vi "FRIC_navX_Internal_Serial_ProcessingLoop.vi"(7 "Device Number":T3, 11 "Rate (4Hz-200Hz)":u8=50 min=4 max=200) -> ()   [LabVIEW 2016]
doc: "This navX VI handles the reading/writing for the navX. All of the good stuff is in here.\nTHIS VI SHOULD NOT BE CALLED BY THE USER!"
uses:
  <vilib>/Rock Robotics/SystemInterfaces/i2clib/i2c_bus.ctl
  TypeDefs/Z900_navX_ProtocolTypeDef.ctl
  navX Library v2.lvlib
  TypeDefs/FRIC_navX_ProcessingLoopStatesTypeDef_I2C.ctl
  TypeDefs/Z900_navX_IntegrationControlRegisters.ctl
  TypeDefs/Z900_navX_ActionTypeDef.ctl
  TypeDefs/Z900_navX_NotifyPacketTypeDef.ctl
  TypeDefs/FRIC_navX_I2C Process Loop TypeDef.ctl
  <vilib>/Rock Robotics/SystemInterfaces/spilib/spi_bus.ctl
  <vilib>/Rock Robotics/WPI/SPI/WPI_SPIDevRef.ctl
  TypeDefs/Z900_navX_SerialStreamTypeDef.ctl
  <vilib>/Rock Robotics/WPI/SerialPort/WPI_SerialPortRef.ctl
  TypeDefs/FRIC_navX_DeviceNumbersTypeDef.ctl
  <vilib>/Rock Robotics/WPI/SerialPort/WPI_SerialPort.ctl
  <vilib>/Platform/TimedLoop/XDataNode/wakeup.ctl
  <vilib>/Platform/TimedLoop/XDataNode/XDNodeRunTimeDep.lvlib
  <vilib>/Platform/TimedLoop/XDataNode/nitl_modes.ctl
  <vilib>/Platform/TimedLoop/XDataNode/timing_clust.ctl
  <vilib>/Platform/TimedLoop/XDataNode/XDataNode.xnode
  <vilib>/ptbypt/NI_PtbyPt.lvlib
  TypeDefs/Z900_navX_DeviceTypeDef.ctl
panel:
  in  "Tab Control":enum32{"Page 1", "Page 2"}(tab)
  in  "Halt":bool
  out "Connected":bool
  out "error":errorcluster
  in  "Stream Type":T1=enum."AHRSAndPositioning"
  in  "Serial Port":T2=enum."MXP TTL"
  out "Loop Time":dbl format="%#.1g"
  out "Loop dt":i64
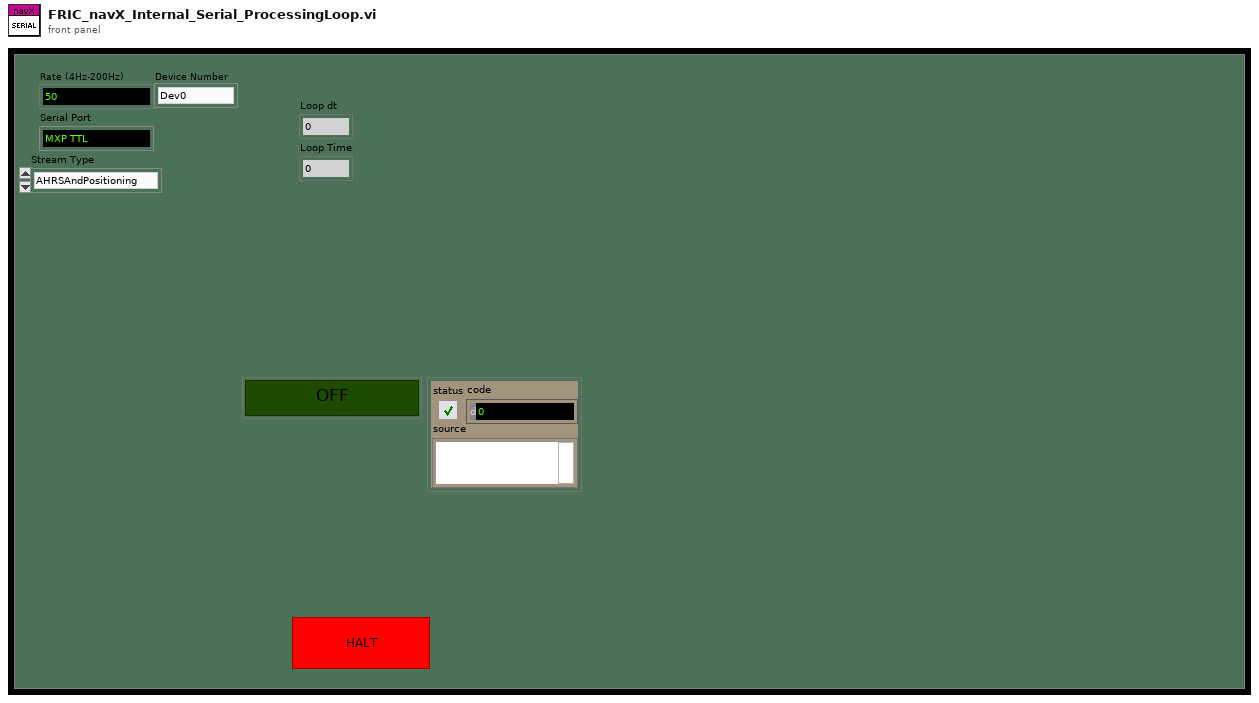
[diagram p1: front panel]
types:
  T1 = typedef "navX Library v2.lvlib/Z900_navX_SerialStreamTypeDef.ctl" = enum16{"YRPH", "Quaterinons", "Gyro/Raw", "AHRS", "AHRSAndPositioning"}
  T2 = typedef "WPI_SerialPort.ctl" = enum16{"Onboard RS-232", "MXP TTL", "USB 1", "USB 2"}
  T3 = typedef "FRIC_navX_DeviceNumbersTypeDef.ctl" = enum16{"Dev0", "Dev1", "Dev2", "Dev3"}
  T4 = typedef "FRIC_navX_I2C Process Loop TypeDef.ctl" = cluster{"State Array":T5[], "error":errorcluster, "FPGA Cluster":cluster{"Last Valid FPGA Time":dbl, "Error Count":i32, "Initialized":bool}, "Device Info":T6, "I2CDevRef":cluster{"DevStatus":errorcluster, "Device Address":u8, "Handle":i32, "I2C Bus":T8}, "Registry":u8[], "Command Array":T9[], "Connected?":bool, "navX Device Memory Size":i32, "notification":T10, "Memory Size Set":bool, "SPIDevRef":T12, "navX Serial Open":cluster{"Stream Type":T1, "Serial Port":T2}, "SerialPortRef":T14, "Serial Read Buffer":string, "Serial Write Buffer":string[], "Device Number":T3, "navX SPI Open":cluster{"SPI Bus":T13, "Clock Rate (Hz)":dbl}, "Loop dt":i64, "current time":timestamp, "Loop Time":i64}
  T5 = typedef "FRIC_navX_ProcessingLoopStatesTypeDef_I2C.ctl" = enum16{"Process", "INI", "Check Packets Valid", "Close", "Flush Serial", "Generate Command", "Last Packet Valid", "Open", "Read", "Reset Serial", "Set Termination Char", "Update AE", "Wait", "Write", "Exit"}
  T6 = typedef "navX Library v2.lvlib/Z900_navX_DeviceTypeDef.ctl" = cluster{"Interface":cluster{"Protocol":T7, "Update Rate (4Hz-100Hz)":u8, "navX Open TypeDef":variant}, "Notify Packet":refnum<notifier>, "Loop VI Refnum":refnum<vi>, "Ready to Close Occurrence Refnum":refnum<k4>}
  T7 = typedef "navX Library v2.lvlib/Z900_navX_ProtocolTypeDef.ctl" = enum16{"SERIAL", "I2C", "SPI"}
  T8 = typedef "i2c_bus.ctl" = enum16{"I2C On-Board", "I2C MXP", "Invalid"}
  T9 = typedef "navX Library v2.lvlib/Z900_navX_IntegrationControlRegisters.ctl" = u8
  T10 = typedef "navX Library v2.lvlib/Z900_navX_NotifyPacketTypeDef.ctl" = cluster{"navX Action":T11, "Data":variant}
  T11 = typedef "navX Library v2.lvlib/Z900_navX_ActionTypeDef.ctl" = enum16{"None", "Halt", "Update Serial Protocol", "Zero-Yaw", "Zero-Displacement", "Zero-Velocity"}
  T12 = typedef "WPI_SPIDevRef.ctl" = cluster{"DevStatus":errorcluster, "Handle":i32, "SPI Bus":T13}
  T13 = typedef "spi_bus.ctl" = enum16{"SPI On-Board, CS0", "SPI On-Board, CS1", "SPI On-Board, CS2", "SPI On-Board, CS3", "SPI MXP", "Invalid"}
  T14 = typedef "WPI_SerialPortRef.ctl" = cluster{"DevStatus":errorcluster, "Serial Port Name":refnum<visa-resource-name>}
  T15 = typedef "XDNodeRunTimeDep.lvlib/timing_clust.ctl" = cluster{"Expected End [f-1]":u64, "Actual End [f-1]":u64, "Finished Late? [f-1]":bool, "Expected End [i-1]":u64, "Actual End [i-1]":u64, "Finished Late? [i-1]":bool, "Expected Start [i]":u64, "Actual Start [i]":u64, "Expected Start [f]":u64, "Actual Start [f]":u64, "Source Name":string, "Structure Name":string, "Period":i64, "Deadline":i64, "Offset":i64, "Start":i64, "Priority":i32, "Timeout":i32, "Mode":T16, "Wakeup Reason":T17, "Error":errorcluster, "Source Type":string, "Secondary Source Type":string, "Global End Time":u64, "Global Start Time":u64, "Frame Duration":u64, "Iteration Duration":u64, "Assigned CPU":i32, "I/O Scan Engine Mode":u32}
  T16 = typedef "XDNodeRunTimeDep.lvlib/nitl_modes.ctl" = enum32{"No Change", "Process missed periods, maintain original phase", "Discard missed periods, maintain original phase", "Process missed periods, ignore original phase", "Discard missed periods, ignore original phase"}
  T17 = typedef "XDNodeRunTimeDep.lvlib/wakeup.ctl" = enum32{"Normal", "Aborted", "Asynchronous wakeup", "Timing source error", "Timed loop error", "Timeout"}
  T18 = typedef "Z900_navX_ActionTypeDef.ctl" = enum16{"None", "Halt", "Normal Read", "Update Serial Protocol", "Update Rate Htz", "Zero-Yaw", "Zero-Displacement", "Zero-Velocity"}
  T19 = cluster{"Last Valid FPGA Time":dbl, "Error Count":i32, "Initialized":bool}
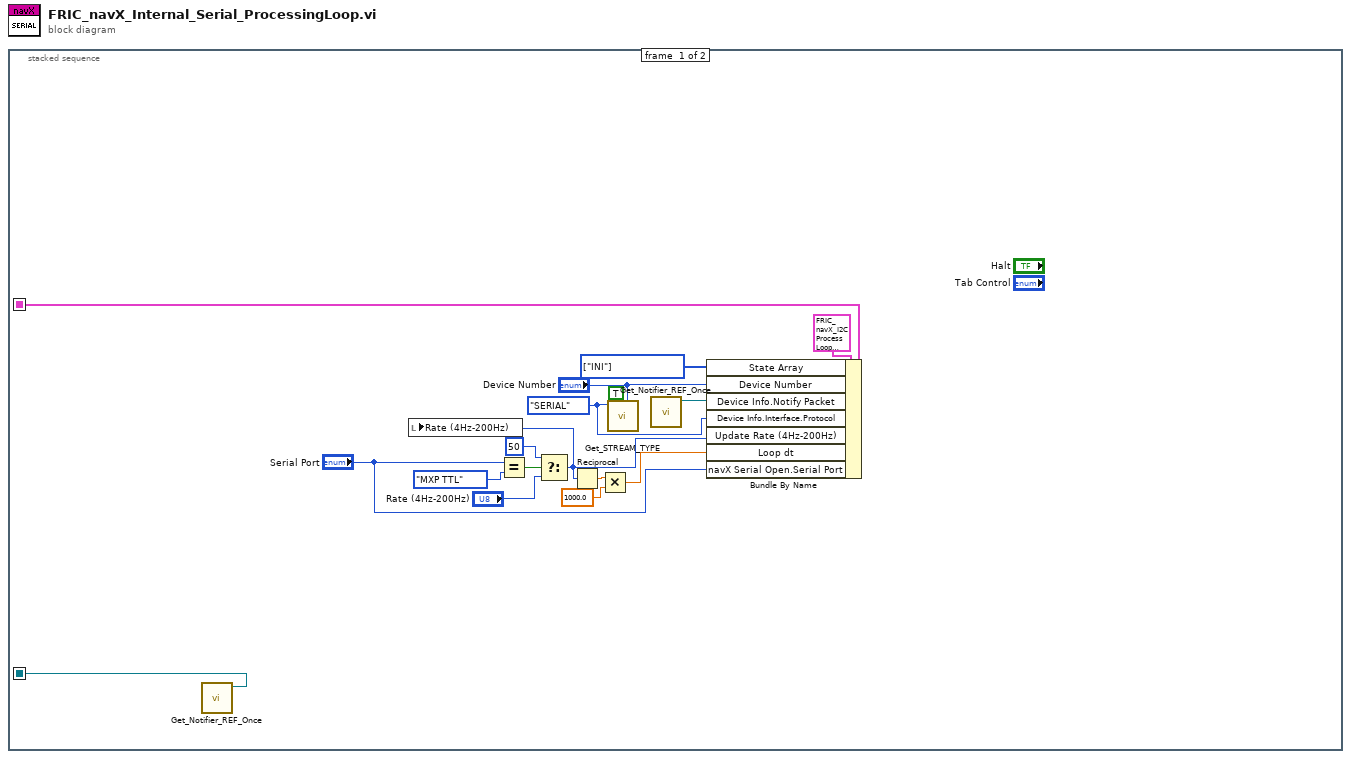
[diagram p0: block diagram]
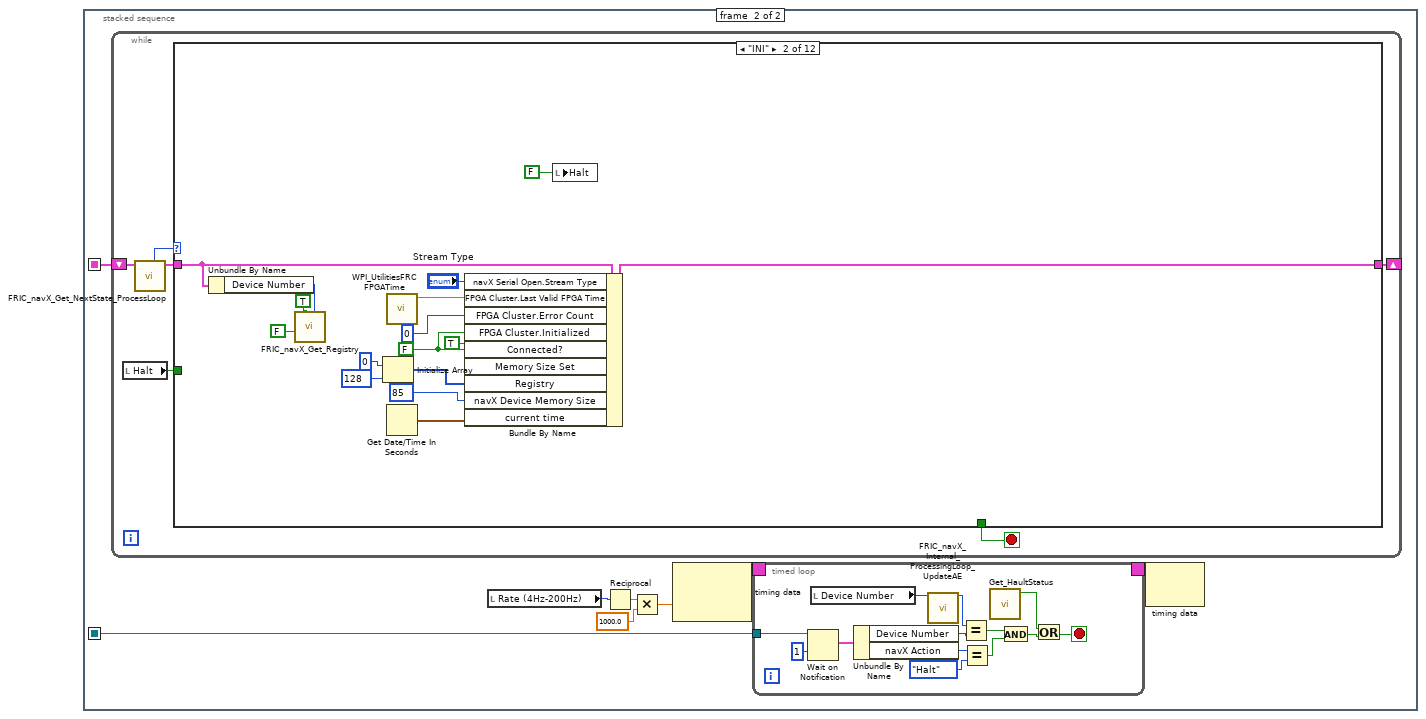
[diagram p2: hidden frame]
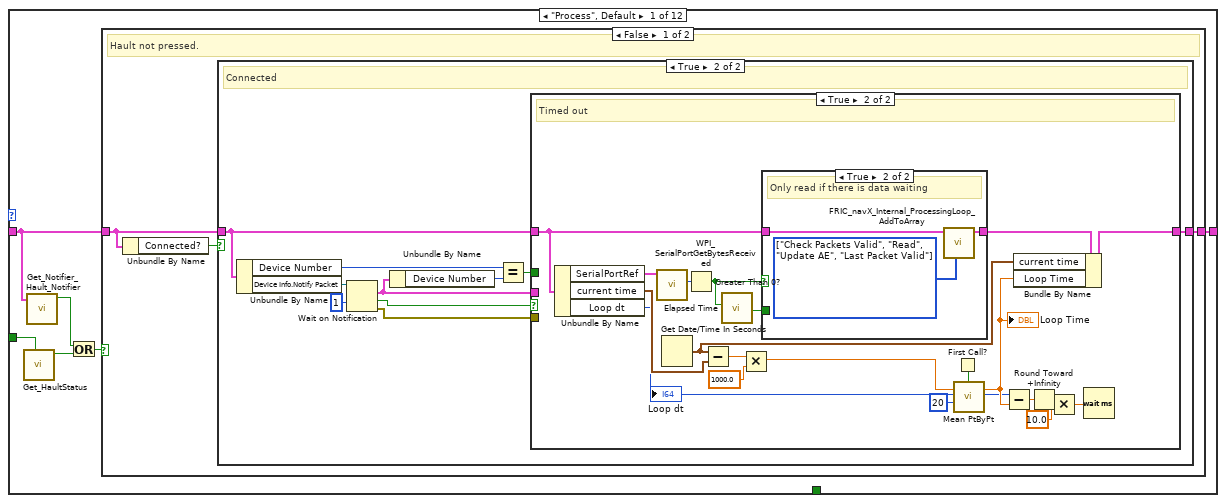
[diagram p3: hidden frame]
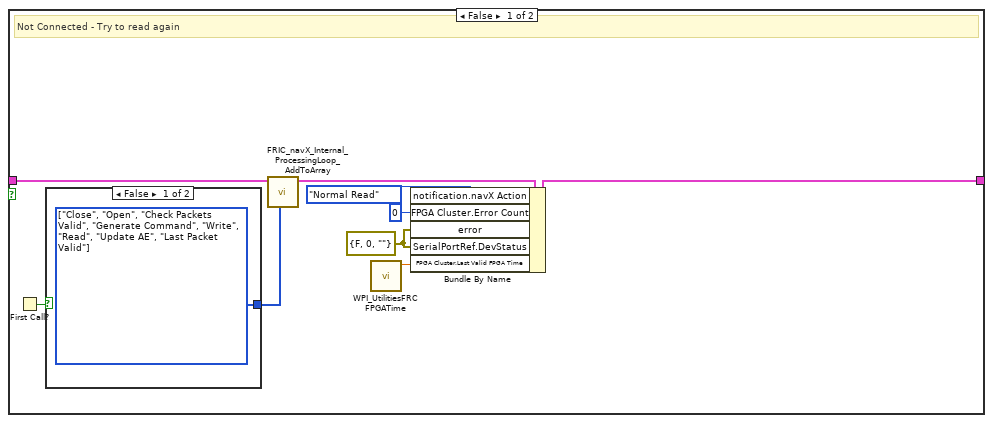
[diagram p4: hidden frame]
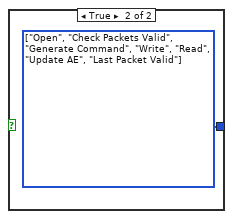
[diagram p5: hidden frame]
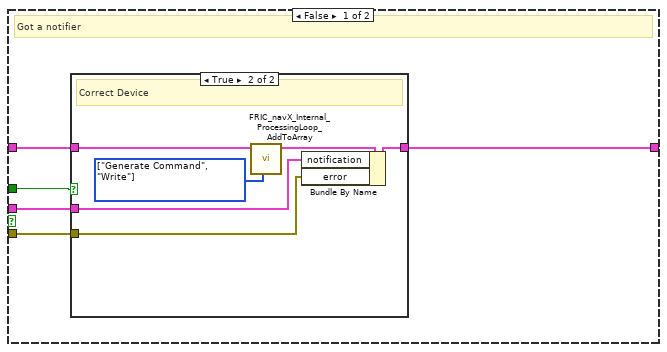
[diagram p6: hidden frame]
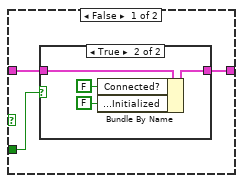
[diagram p8: hidden frame]
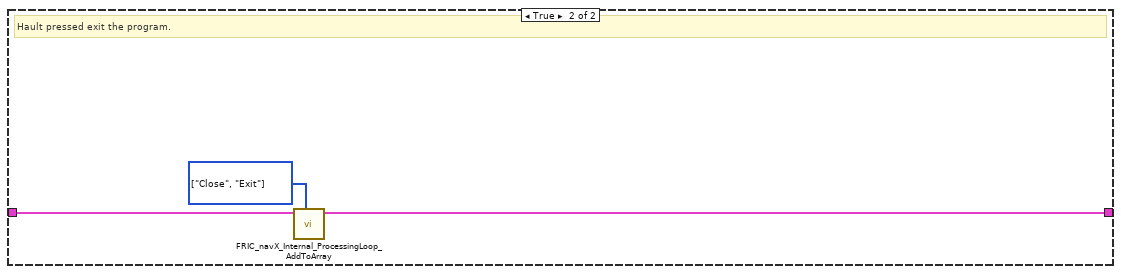
[diagram p10: hidden frame]
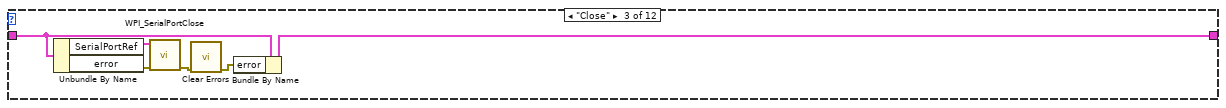
[diagram p11: hidden frame]
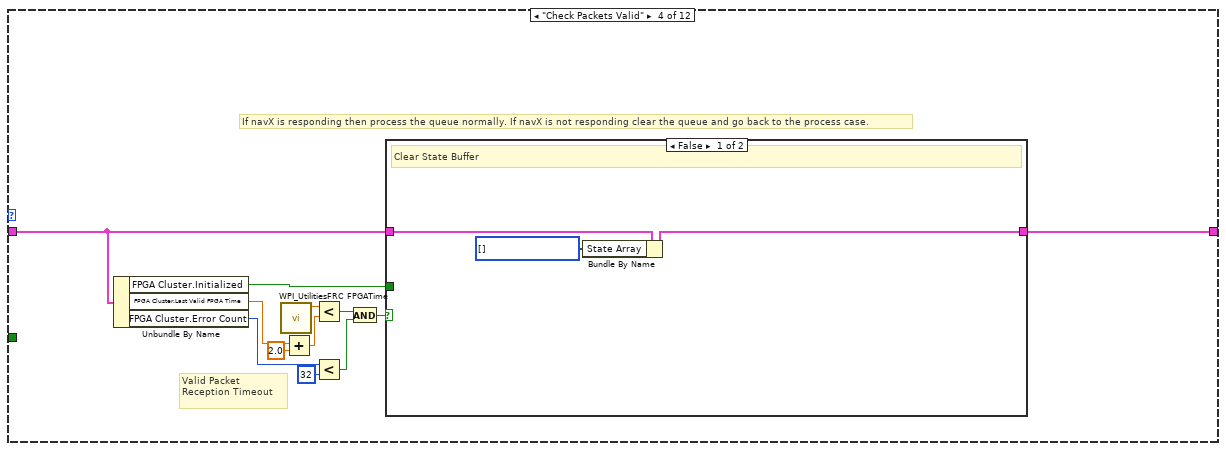
[diagram p12: hidden frame]
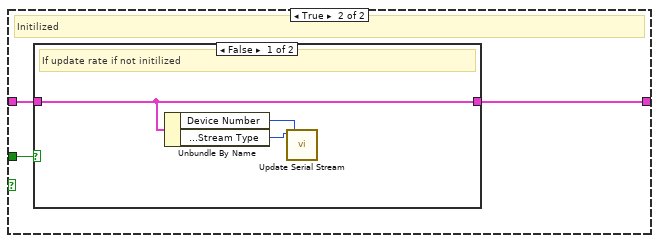
[diagram p13: hidden frame]
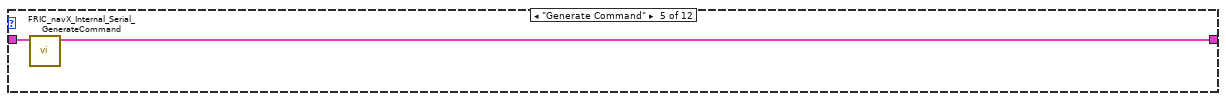
[diagram p15: hidden frame]
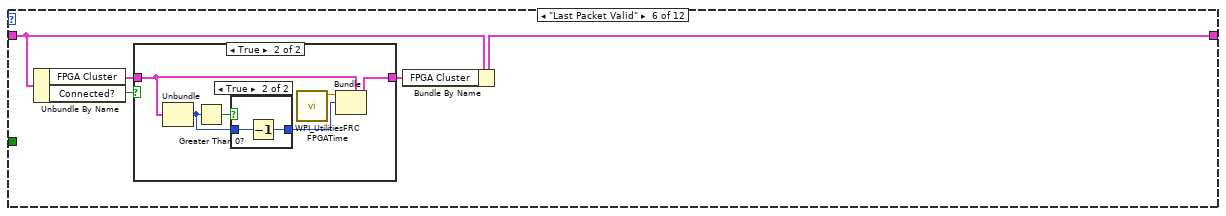
[diagram p16: hidden frame]
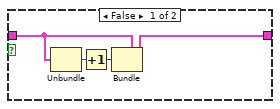
[diagram p17: hidden frame]
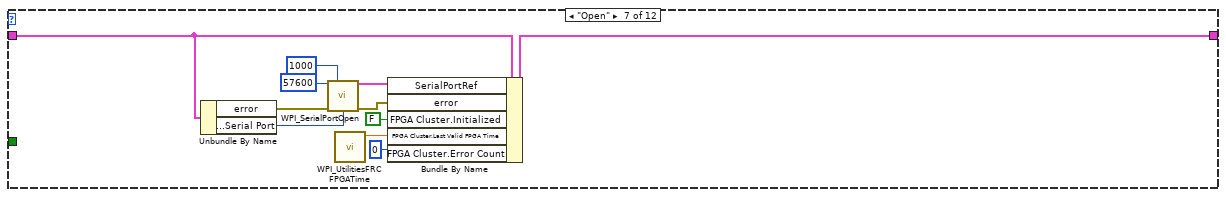
[diagram p19: hidden frame]
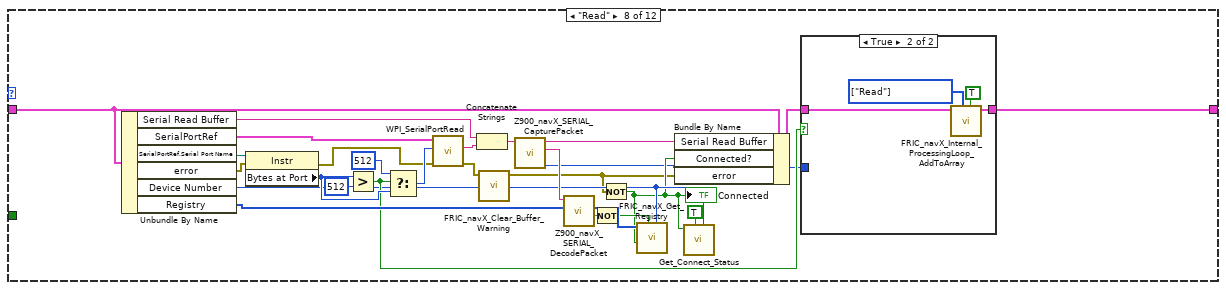
[diagram p20: hidden frame]
diagram:
  n1 = stacked-sequence {
    seq-local: [w17 _] -> [_ w25]
    seq-local: [w13 _] -> [_ w18]
    frame #0 {
      w1 = Z900_navX_ProtocolTypeDef."SERIAL" ("Protocol")
      w15 = T5[] [enum."INI"] items=["Process", "INI", "Check Packets Valid", "Close", "Flush Serial", "Generate Command", "Last Packet Valid", "Open", "Read", "Reset Serial", "Set Termination Char", "Update AE", "Wait", "Write", "Exit"] ("State Array")
      n2 = call "Get_Notifier_REF_Once.vi"() -> ("notifier ref out"=w13:refnum<notifier>)  [unwired: 10 in, 1 out]
      n3 = Equal?(x="Serial Port", y=WPI_SerialPort."MXP TTL") -> (x = y?=w11:bool)
      n4 = Select(t=u8 50, s=w11, f="Rate (4Hz-200Hz)") -> (s? t:f=w6:u8)
      n5 = local write "Rate (4Hz-200Hz)"(w6) -> ()
      n6 = Reciprocal(x=w6) -> (1/x=w9:dbl)
      n7 = Multiply(x=w9, y=1000.0) -> (x*y=w7:dbl)
      n8 = call "Get_STREAM_TYPE.vi"("Device Number"="Device Number", "Update"=TRUE, "Protocol (in)"=w1) -> ()  [unwired: 8 in, 1 out]
      n9 = call "Get_Notifier_REF_Once.vi"() -> ("notifier ref out"=w14:refnum<notifier>)  [unwired: 10 in, 1 out]
      n10 = Bundle By Name(cluster=T4 {"State Array"=[enum."INI", enum."Open"], "error"={"status"=FALSE, "code"=0, "source"=""}, "FPGA Cluster"={"Last Valid FPGA Time"=0.0, "Error Count"=0, "Initialized"=FALSE}, "Device Info"={"Interface"={"Protocol"=enum."SERIAL", "Update Rate (4Hz-100Hz)"=4, "navX Open TypeDef"=variant}, "Notify Packet"=refnum, "Loop VI Refnum"=refnum, "Ready to Close Occurrence Refnum"=refnum}, "I2CDevRef"={"DevStatus"={"status"=FALSE, "code"=0, "source"=""}, "Device Address"=0, "Handle"=0, "I2C Bus"=enum."Invalid"}, "Registry"=[], "Command Array"=[214, 32], "Connected?"=FALSE, "navX Device Memory Size"=85, "notification"={"navX Action"=enum."None", "Data"=variant}, "Memory Size Set"=FALSE, "SPIDevRef"={"DevStatus"={"status"=FALSE, "code"=0, "source"=""}, "Handle"=0, "SPI Bus"=enum."SPI On-Board, CS0"}, "navX Serial Open"={"Stream Type"=enum."YRPH", "Serial Port"=enum."Onboard RS-232"}, "SerialPortRef"={"DevStatus"={"status"=FALSE, "code"=0, "source"=""}, "Serial Port Name"=""}, "Serial Read Buffer"="", "Serial Write Buffer"=[], "Device Number"=enum."Dev0", "navX SPI Open"={"SPI Bus"=enum."SPI MXP", "Clock Rate (Hz)"=500000.0}, "Loop dt"=0, "current time"=timestamp(0 s since 1904-01-01), "Loop Time"=0} ("I2C Process Loop TypeDef"), "State Array"=w15, "Device Number"="Device Number", "Device Info.Notify Packet"=w14, "Device Info.Interface.Protocol"=w1, "Update Rate (4Hz-200Hz)"=w6, "Loop dt"=w7, "navX Serial Open.Serial Port"="Serial Port") -> (w17:T4)
    }
    frame #1 {
      n11 = while {
        shift-right: [w45] -> _
        shift-left: w25 -> [w48]
        stop <- w49 stop-if-true
        n12 = local read "Halt"() -> (w44:bool)
        n13 = call "FRIC_navX_Get_NextState_ProcessLoop.vi"("I2C Process Loop TypeDef (in)"=w48) -> ("I2C Process Loop TypeDef (out)"=w47:T4, "Current State"=w46:T5)  [unwired: 9 in]
        n14 = case shown="\"INI\"" w46 {
          tunnel: [_ _ _ _ _ _ _ _ _ _ TRUE _] -> w49
          tunnel: w47 -> [w53 w130 w147 w151 w171 w175 w200 w212 w237 w250 w257 w265]
          tunnel: [w55 w137 w146 w152 w170 w174 w199 w209 w238 w239 w257 w265] -> w45
          tunnel: w44 -> [w54 _ _ _ _ _ _ _ _ _ _ _]
          frame "Process", Default {
            n15 = call "Get_HaultStatus.vi"("Update"=w54) -> ("Hault"=w51:bool)  [unwired: 10 in]
            n16 = call "Get_Notifier_Hault_Notifier.vi"("Process Loop TypeDef (in)"=w53) -> ("Hault Notifier"=w52:bool)  [unwired: 10 in]
            n17 = Or(x=w52, y=w51) -> (x .or. y?=w50:bool)
            n18 = case shown="False" w50 {
              tunnel: [w58 w124] -> w55
              tunnel: w53 -> [w56 w125]
              frame False {
                # "Hault not pressed."
                n19 = Unbundle By Name(w56) -> ("Connected?"=w57:bool)
                n20 = case shown="True" w57 {
                  tunnel: w56 -> [w67 w78]
                  tunnel: [w64 w79] -> w58
                  frame False {
                    w60 = errorcluster {"status"=FALSE, "code"=0, "source"=""} ("error")
                    # "Not Connected - Try to read again"
                    n21 = First Call?() -> (First Call?: T/F=w61:bool)
                    n22 = case shown="False" w61 {
                      tunnel: [w68 w69] -> w66
                      frame False {
                        w68 = T5[] [enum."Close", enum."Open", enum."Check Packets Valid", enum."Generate Command", enum."Write", enum."Read", enum."Update AE", enum."Last Packet Valid"] items=["Process", "INI", "Check Packets Valid", "Close", "Flush Serial", "Generate Command", "Last Packet Valid", "Open", "Read", "Reset Serial", "Set Termination Char", "Update AE", "Wait", "Write", "Exit"]
                      }
                      frame True {
                        w69 = T5[] [enum."Open", enum."Check Packets Valid", enum."Generate Command", enum."Write", enum."Read", enum."Update AE", enum."Last Packet Valid"] items=["Process", "INI", "Check Packets Valid", "Close", "Flush Serial", "Generate Command", "Last Packet Valid", "Open", "Read", "Reset Serial", "Set Termination Char", "Update AE", "Wait", "Write", "Exit"]
                      }
                    }
                    n23 = call "FRIC_navX_Internal_ProcessingLoop_AddToArray.vi"("States Array"=w66, "I2C Process Loop TypeDef (in)"=w67) -> ("I2C Process Loop TypeDef (out)"=w65:T4)  [unwired: 9 in]
                    n24 = call <vilib>:"WPI_UtilitiesFRC FPGATime.vi"() -> ("FPGA Time"=w59:dbl)  [unwired: 10 in, 1 out]
                    n25 = Bundle By Name(cluster=w65, "notification.navX Action"=Z900_navX_ActionTypeDef."Normal Read", "FPGA Cluster.Error Count"=0, "error"=w60, "SerialPortRef.DevStatus"=w60, "FPGA Cluster.Last Valid FPGA Time"=w59) -> (w64:T4)
                  }
                  frame True {
                    # "Connected"
                    n26 = Unbundle By Name(w78) -> ("Device Number"=w72:T3, "Device Info.Notify Packet"=w77:refnum<notifier>)
                    n27 = Wait on Notification(notifier=w77, timeout in ms (-1)=1) -> (notification=w73:T10, timed out?=w74:bool, error out=w75:errorcluster)  [unwired: 2 in, 1 out]
                    n28 = Unbundle By Name(w73) -> ("Device Number"=w71:T3)
                    n29 = Equal?(x=w72, y=w71) -> (x = y?=w70:bool)
                    n30 = case shown="True" w74 {
                      tunnel: w78 -> [w84 w108]
                      tunnel: [w83 w102] -> w79
                      tunnel: w73 -> [w82 _]
                      tunnel: w75 -> [w81 _]
                      tunnel: w70 -> [w80 _]
                      frame False {
                        # "Got a notifier"
                        n31 = case shown="True" w80 {
                          tunnel: w84 -> [w85 w91]
                          tunnel: [w85 w90] -> w83
                          tunnel: w82 -> [_ w89]
                          tunnel: w81 -> [_ w86]
                          frame False {
                          }
                          frame True {
                            w87 = T5[] [enum."Generate Command", enum."Write"] items=["Process", "INI", "Check Packets Valid", "Close", "Flush Serial", "Generate Command", "Last Packet Valid", "Open", "Read", "Reset Serial", "Set Termination Char", "Update AE", "Wait", "Write", "Exit"] ("States Array")
                            # "Correct Device"
                            n32 = call "FRIC_navX_Internal_ProcessingLoop_AddToArray.vi"("States Array"=w87, "I2C Process Loop TypeDef (in)"=w91) -> ("I2C Process Loop TypeDef (out)"=w88:T4)  [unwired: 9 in]
                            n33 = Bundle By Name(cluster=w88, "notification"=w89, "error"=w86) -> (w90:T4)
                          }
                        }
                      }
                      frame True {
                        # "Timed out"
                        n34 = Unbundle By Name(w108) -> ("SerialPortRef"=w110:T14, "current time"=w105:timestamp, "Loop dt"=w93:i64)
                        "Loop dt" <- w93
                        n35 = call <vilib>:"WPI_SerialPortGetBytesReceived.vi"("SerialPortRef"=w110) -> ("Bytes at Port"=w109:u32)  [unwired: 8 in, 2 out]
                        n36 = Get Date/Time In Seconds() -> (seconds since 1Jan1904=w101:timestamp)
                        n37 = Greater Than 0?(x=w109) -> (x > 0?=w107:bool)
                        n38 = Subtract(x=w101, y=w105) -> (x-y=w104:dbl)
                        n39 = call "Elapsed Time"("Reset"=w107) -> ("Time has Elapsed"=w106:bool)  [unwired: 11 in, 7 out]
                        n40 = Multiply(x=w104, y=1000.0) -> (x*y=w95:dbl)
                        n41 = case shown="True" w107 {
                          tunnel: [w112 w121] -> w111
                          tunnel: w108 -> [w113 w120]
                          tunnel: w106 -> [w114 _]
                          frame False {
                            n42 = case shown="True" w114 {
                              tunnel: w113 -> [w115 w119]
                              tunnel: [w115 w118] -> w112
                              frame False {
                              }
                              frame True {
                                n43 = Bundle By Name(cluster=w119, "Connected?"=FALSE, "FPGA Cluster.Initialized"=FALSE) -> (w118:T4)
                              }
                            }
                          }
                          frame True {
                            w122 = T5[] [enum."Check Packets Valid", enum."Read", enum."Update AE", enum."Last Packet Valid"] items=["Process", "INI", "Check Packets Valid", "Close", "Flush Serial", "Generate Command", "Last Packet Valid", "Open", "Read", "Reset Serial", "Set Termination Char", "Update AE", "Wait", "Write", "Exit"]
                            # "Only read if there is data waiting"
                            n44 = call "FRIC_navX_Internal_ProcessingLoop_AddToArray.vi"("States Array"=w122, "I2C Process Loop TypeDef (in)"=w120) -> ("I2C Process Loop TypeDef (out)"=w121:T4)  [unwired: 9 in]
                          }
                        }
                        n45 = First Call?() -> (First Call?: T/F=w96:bool)
                        n46 = call <vilib>:"Mean PtByPt.vi"("x"=w95, "sample length"=20, "initialize"=w96) -> ("mean"=w94:dbl)  [unwired: 1 in, 1 out]
                        "Loop Time" <- w94
                        n47 = Subtract(x=w93, y=w94) -> (x-y=w98:dbl)
                        n48 = Bundle By Name(cluster=w111, "current time"=w101, "Loop Time"=w94) -> (w102:T4)
                        n49 = Round Toward +Infinity(x=w98) -> (ceil(x): smallest int >= x=w100:dbl)
                        n50 = Multiply(x=w100, y=10.0) -> (x*y=w92:dbl)
                        n51 = Wait (ms)(milliseconds to wait=w92) -> ()  [unwired: 1 out]
                      }
                    }
                  }
                }
              }
              frame True {
                w123 = T5[] [enum."Close", enum."Exit"] items=["Process", "INI", "Check Packets Valid", "Close", "Flush Serial", "Generate Command", "Last Packet Valid", "Open", "Read", "Reset Serial", "Set Termination Char", "Update AE", "Wait", "Write", "Exit"] ("States Array")
                # "Hault pressed exit the program."
                n52 = call "FRIC_navX_Internal_ProcessingLoop_AddToArray.vi"("States Array"=w123, "I2C Process Loop TypeDef (in)"=w125) -> ("I2C Process Loop TypeDef (out)"=w124:T4)  [unwired: 9 in]
              }
            }
          }
          frame "INI" {
            w135 = FALSE ("Initialized")
            n53 = Unbundle By Name(w130) -> ("Device Number"=w129:T3)
            n54 = call "FRIC_navX_Get_Registry.vi"("Device Number"=w129, "Update"=TRUE, "Connected?"=FALSE) -> ()  [unwired: 7 in, 2 out]
            n55 = Initialize Array(u8 0 ("Received Data"), 128 ("hex")) -> (w133:u8[])
            n56 = call <vilib>:"WPI_UtilitiesFRC FPGATime.vi"() -> ("FPGA Time"=w139:dbl)  [unwired: 10 in, 1 out]
            n57 = Get Date/Time In Seconds() -> (seconds since 1Jan1904=w126:timestamp)
            n58 = Bundle By Name(cluster=w130, "navX Serial Open.Stream Type"="Stream Type", "FPGA Cluster.Last Valid FPGA Time"=w139, "FPGA Cluster.Error Count"=0 ("Error Count"), "FPGA Cluster.Initialized"=w135, "Connected?"=w135, "Memory Size Set"=TRUE, "Registry"=w133, "navX Device Memory Size"=85 ("hex"), "current time"=w126) -> (w137:T4)
            n59 = local write "Halt"(FALSE ("Halt")) -> ()
          }
          frame "Close" {
            n60 = Unbundle By Name(w147) -> ("SerialPortRef"=w144:T14, "error"=w143:errorcluster)
            n61 = call <vilib>:"WPI_SerialPortClose.vi"("error in (no error)"=w143, "SerialPortRef"=w144) -> ("error out"=w142:errorcluster)  [unwired: 9 in]
            n62 = call <vilib>:"Clear Errors.vi"("error in (no error)"=w142) -> ("error out"=w145:errorcluster)  [unwired: 5 in, 1 out]
            n63 = Bundle By Name(cluster=w147, "error"=w145) -> (w146:T4)
          }
          frame "Check Packets Valid" {
            # "If navX is responding then process the queue normally. If navX is not responding clear the queue and go back to the process case."
            # "Valid Packet Reception Timeout"
            n64 = Unbundle By Name(w151) -> ("FPGA Cluster.Initialized"=w149:bool, "FPGA Cluster.Last Valid FPGA Time"=w150:dbl, "FPGA Cluster.Error Count"=w148:i32)
            n65 = call <vilib>:"WPI_UtilitiesFRC FPGATime.vi"() -> ("FPGA Time"=w157:dbl)  [unwired: 10 in, 1 out]
            n66 = Add(x=w150, y=2.0) -> (x+y=w158:dbl)
            n67 = Less?(x=w157, y=w158) -> (x < y?=w155:bool)
            n68 = Less?(x=w148, y=32) -> (x < y?=w154:bool)
            n69 = And(x=w155, y=w154) -> (x .and. y?=w153:bool)
            n70 = case shown="False" w153 {
              tunnel: w151 -> [w162 w165]
              tunnel: [w161 w164] -> w152
              tunnel: w149 -> [_ w163]
              frame False {
                w160 = T5[] [] items=["Process", "INI", "Check Packets Valid", "Close", "Flush Serial", "Generate Command", "Last Packet Valid", "Open", "Read", "Reset Serial", "Set Termination Char", "Update AE", "Wait", "Write", "Exit"] ("f")
                # "Clear State Buffer"
                n71 = Bundle By Name(cluster=w162, "State Array"=w160) -> (w161:T4)
              }
              frame True {
                # "Initilized"
                n72 = case shown="False" w163 {
                  tunnel: w165 -> [w168 w169]
                  tunnel: [w168 w169] -> w164
                  frame False {
                    # "If update rate if not initilized"
                    n73 = Unbundle By Name(w168) -> ("Device Number"=w167:T3, "navX Serial Open.Stream Type"=w166:T1)
                    n74 = call "Update Serial Stream.vi"("Device Number"=w167, "Stream Type"=w166) -> ()  [unwired: 10 in]
                  }
                  frame True {
                    # "Everything is good keep going"
                  }
                }
              }
            }
          }
          frame "Generate Command" {
            n75 = call "FRIC_navX_Internal_Serial_GenerateCommand.vi"("Serial Process Loop TypeDef (in)"=w171) -> ("Serial Process Loop TypeDef (out)"=w170:T4)  [unwired: 10 in]
          }
          frame "Last Packet Valid" {
            n76 = Unbundle By Name(w175) -> ("FPGA Cluster"=w176:T19, "Connected?"=w172:bool)
            n77 = case shown="True" w172 {
              tunnel: [w179 w186] -> w173
              tunnel: w176 -> [w178 w182]
              frame False {
                n78 = Unbundle(w178) -> ("Error Count"=w177:i32)  [unwired: 2 out]
                n79 = Increment(x=w177) -> (x+1=w180:i32)
                n80 = Bundle(cluster=w178, "Error Count"=w180) -> (w179:T19)  [unwired: 2 in]
              }
              frame True {
                n81 = Unbundle(w182) -> ("Error Count"=w181:i32)  [unwired: 2 out]
                n82 = Greater Than 0?(x=w181) -> (x > 0?=w184:bool)
                n83 = case shown="True" w184 {
                  tunnel: [w187 w189] -> w183
                  tunnel: w181 -> [w187 w188]
                  frame False {
                  }
                  frame True {
                    n84 = Decrement(x=w188) -> (x-1=w189:i32)
                  }
                }
                n85 = call <vilib>:"WPI_UtilitiesFRC FPGATime.vi"() -> ("FPGA Time"=w185:dbl)  [unwired: 10 in, 1 out]
                n86 = Bundle(cluster=w182, "Last Valid FPGA Time"=w185, "Error Count"=w183) -> (w186:T19)  [unwired: 1 in]
              }
            }
            n87 = Bundle By Name(cluster=w175, "FPGA Cluster"=w173) -> (w174:T4)
          }
          frame "Open" {
            n88 = Unbundle By Name(w200) -> ("error"=w191:errorcluster, "navX Serial Open.Serial Port"=w190:T2)
            n89 = call <vilib>:"WPI_SerialPortOpen.vi"("Baud Rate"=u32 57600, "Timeout Value (ms)"=u32 1000, "error in (no error)"=w191, "Serial Port"=w190) -> ("SerialPortRef"=w194:T14, "error out"=w195:errorcluster)  [unwired: 10 in]
            n90 = call <vilib>:"WPI_UtilitiesFRC FPGATime.vi"() -> ("FPGA Time"=w193:dbl)  [unwired: 10 in, 1 out]
            n91 = Bundle By Name(cluster=w200, "SerialPortRef"=w194, "error"=w195, "FPGA Cluster.Initialized"=FALSE ("Initialized"), "FPGA Cluster.Last Valid FPGA Time"=w193, "FPGA Cluster.Error Count"=0) -> (w199:T4)
          }
          frame "Read" {
            n92 = Unbundle By Name(w212) -> ("Serial Read Buffer"=w223:string, "SerialPortRef"=w224:T14, "SerialPortRef.Serial Port Name"=w227:refnum<visa-resource-name>, "error"=w226:errorcluster, "Device Number"=w207:T3, "Registry"=w214:u8[])
            n93 = property class="Instr"(reference=w227, error in=w226) -> (error out=w217:errorcluster, "Bytes at Port"=w220:u32)  [unwired: 1 in]
            n94 = Greater?(x=w220, y=u32 512) -> (0:w208:bool)
            n95 = Select(t=u32 512 ("y"), s=w208, f=w220) -> (s? t:f=w218:u32)
            n96 = call <vilib>:"WPI_SerialPortRead.vi"("error in (no error)"=w217, "Num Bytes to Read"=w218, "SerialPortRef"=w224) -> ("error out"=w202:errorcluster, "Buffer"=w225:string)  [unwired: 6 in, 1 out]
            n97 = Concatenate Strings(w223, w225) -> (w222:string)
            n98 = call "FRIC_navX_Clear_Buffer_Warning.vi"("error in"=w202) -> ("error out"=w201:errorcluster)  [unwired: 10 in]
            n99 = call "Z900_navX_SERIAL_CapturePacket.vi"("Buffer"=w222) -> ("Packet Size"=w203:i32, "Packet"=w213:string, "Buffer"=w216:string)  [unwired: 7 in, 1 out]
            n100 = call "Z900_navX_SERIAL_DecodePacket.vi"("Data"=w214, "Packet"=w213) -> (1:w206, "Data"=w215:u8[])  [unwired: 6 in, 2 out]
            n101 = Not(x=w206) -> (.not. x?=w205:bool)
            n102 = Not(x=w201) -> (.not. x?=w204:bool)
            "Connected" <- w204
            n103 = call "FRIC_navX_Get_Registry.vi"("Device Number"=w207, "Update"=w205, "Connected?"=w204, "Registry (in)"=w215) -> ()  [unwired: 6 in, 2 out]
            n104 = Bundle By Name(cluster=w212, "Serial Read Buffer"=w216, "Connected?"=w204, "error"=w201) -> (w210:T4)
            n105 = call "Get_Connect_Status.vi"("Device Number"=w207, "Update"=TRUE, "Connected"=w204) -> ()  [unwired: 8 in, 1 out]
            n106 = case shown="True" w208 {
              tunnel: w210 -> [w228 w232]
              tunnel: [w228 w231] -> w209
              tunnel: w203 -> [_ _]
              frame False {
              }
              frame True {
                w230 = T5[] [enum."Read"] items=["Process", "INI", "Check Packets Valid", "Close", "Flush Serial", "Generate Command", "Last Packet Valid", "Open", "Read", "Reset Serial", "Set Termination Char", "Update AE", "Wait", "Write", "Exit"] ("States Array")
                n107 = call "FRIC_navX_Internal_ProcessingLoop_AddToArray.vi"("Add to beginning"=TRUE, "States Array"=w230, "I2C Process Loop TypeDef (in)"=w232) -> ("I2C Process Loop TypeDef (out)"=w231:T4)  [unwired: 8 in]
              }
            }
          }
          frame "Reset Serial" {
            n108 = Unbundle By Name(w237) -> ("SerialPortRef"=w236:T14, "error"=w234:errorcluster)
            n109 = call <vilib>:"WPI_SerialPortReset.vi"("error in (no error)"=w234, "SerialPortRef"=w236) -> ("error out"=w233:errorcluster, "SerialPortRef"=w235:T14)  [unwired: 8 in]
            n110 = Bundle By Name(cluster=w237, "SerialPortRef"=w235, "error"=w233) -> (w238:T4)
          }
          frame "Write" {
            n111 = Unbundle By Name(w250) -> ("SerialPortRef"=w248:T14, "Serial Write Buffer"=w245:string[], "SerialPortRef.DevStatus"=w249:errorcluster)
            n112 = Delete From Array(array=w245, index=0) -> (deleted portion=w244:string, array with subset deleted=w241:string[])  [unwired: 1 in]
            n113 = call <vilib>:"WPI_SerialPortWrite.vi"("error in (no error)"=w249, "Buffer"=w244, "SerialPortRef"=w248) -> ("error out"=w247:errorcluster, "SerialPortRef"=w246:T14)  [unwired: 6 in, 1 out]
            n114 = Empty Array?(array=w241) -> (empty?=w240:bool)
            n115 = Bundle By Name(cluster=w250, "SerialPortRef"=w246, "error"=w247, "Serial Write Buffer"=w241) -> (w242:T4)
            n116 = case shown="False" w240 {
              tunnel: [w254 w255] -> w239
              tunnel: w242 -> [w253 w255]
              frame False {
                w252 = T5[] [enum."Write"] items=["Process", "INI", "Check Packets Valid", "Close", "Flush Serial", "Generate Command", "Last Packet Valid", "Open", "Read", "Reset Serial", "Set Termination Char", "Update AE", "Wait", "Write", "Exit"] ("States Array")
                # "Write again because buffer is not empty."
                n117 = call "FRIC_navX_Internal_ProcessingLoop_AddToArray.vi"("Add to beginning"=TRUE, "States Array"=w252, "I2C Process Loop TypeDef (in)"=w253) -> ("I2C Process Loop TypeDef (out)"=w254:T4)  [unwired: 8 in]
              }
              frame True {
                # "Process the rest of the state array"
              }
            }
          }
          frame "Exit" {
            n118 = Unbundle By Name(w257) -> ("Device Info"=w256:T6)
            n119 = in-place {
              in-place-border: w256 -> [w260]
              # "Set Occurence of Close"
              n120 = Unbundle By Name(w260) -> ("Ready to Close Occurrence Refnum"=w261:refnum<k4>)
              n121 = local write "Halt"(FALSE ("Halt")) -> ()
              n122 = Set Occurrence(w261) -> ()
            }
          }
          frame "Update AE" {
            n123 = Unbundle By Name(w265) -> ("Device Number"=w263:T3, "error"=w264:errorcluster)
            "error" <- w264
            n124 = call "Get_Error_Status.vi"("Device Number"=w263, "Update"=TRUE, "error in"=w264) -> ()  [unwired: 8 in, 1 out]
          }
        }
      }
      n125 = local read "Rate (4Hz-200Hz)"() -> (w23:u8)
      n126 = Reciprocal(x=w23) -> (1/x=w22:dbl)
      n127 = Multiply(x=w22, y=1000.0) -> (x*y=w19:dbl)
      n128 = node-c288(w19) -> (w21:T15)  [unwired: 1 in]
      n129 = timed-loop {
        timing: w21 -> [_]
        timing-out: [_] -> w20
        tunnel: w18 -> [w29]
        stop <- w28 stop-if-true
        n130 = Wait on Notification(notifier=w29, timeout in ms (-1)=1) -> (notification=w34:T10)  [unwired: 2 in, 3 out]
        n131 = local read "Device Number"() -> (w32:T3)
        n132 = Unbundle By Name(w34) -> ("Device Number"=w33:T3, "navX Action"=w36:T11)
        n133 = call "FRIC_navX_Internal_ProcessingLoop_UpdateAE.vi"("Device Number"=w32) -> ()  [unwired: 15 in]
        n134 = Equal?(x=w32, y=w33) -> (x = y?=w31:bool)
        n135 = Equal?(x=w36, y=Z900_navX_ActionTypeDef."Halt") -> (x = y?=w30:bool)
        n136 = call "Get_HaultStatus.vi"() -> ("Hault"=w27:bool)  [unwired: 11 in]
        n137 = And(x=w31, y=w30) -> (x .and. y?=w26:bool)
        n138 = Or(x=w27, y=w26) -> (x .or. y?=w28:bool)
      }
      n139 = node-c288(w20) -> ()  [unwired: 1 out]
    }
  }
